vi "Read Configuration.vi"(8 "error in (no error)":errorcluster, 11 "RandomNumberGenerator Controller in":refnum<class "RandomNumberGenerator Controller.lvclass">) -> (0 "error out":errorcluster, 2 "Configuration":T1, 3 "RandomNumberGenerator Controller out":refnum<class "RandomNumberGenerator Controller.lvclass">)   [LabVIEW 2020, in "RandomNumberGenerator.lvlib" / "RandomNumberGenerator Controller.lvclass"]
doc: "<b>Read Configuration</b>\nThis method directly returns the <b>Configuration.ct</b> stored in the class data of this plugin's controller."
uses:
  RandomNumberGenerator Controller.lvclass
  RandomNumberGenerator Controller.lvclass/RandomNumberGenerator Controller.ctl
  PE/Configuration.ctl
  PE/RandomNumberGenerator.lvclass
panel:
  # "#via_ignore"
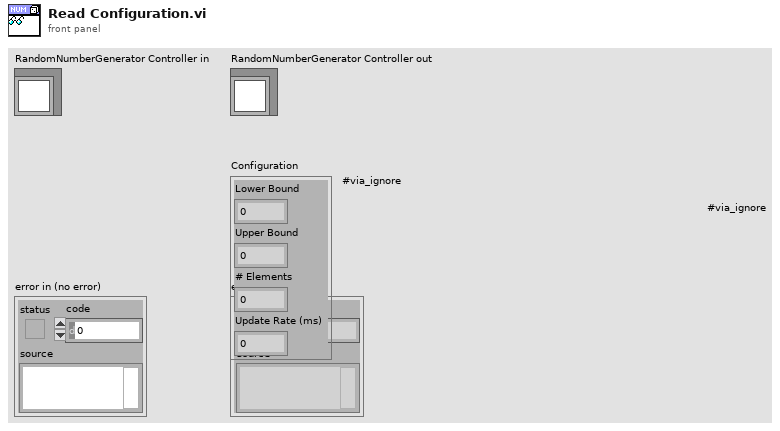
[diagram p1: front panel]
types:
  T1 = typedef "RandomNumberGenerator.lvlib/RandomNumberGenerator.lvclass/Configuration.ctl" = cluster{"Lower Bound":dbl, "Upper Bound":dbl, "# Elements":i32, "Update Rate (ms)":i32}
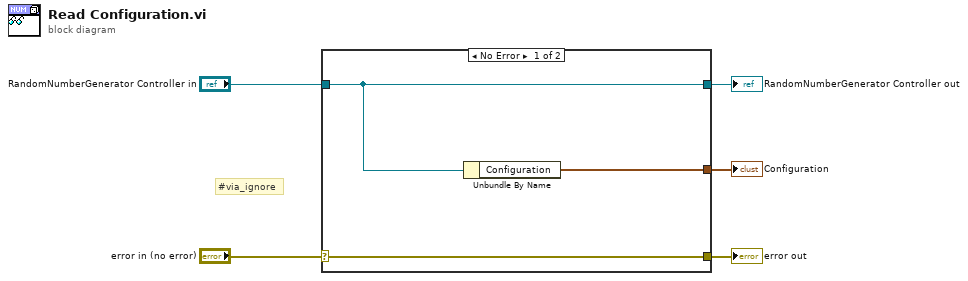
[diagram p0: block diagram]
diagram:
  # "#via_ignore"
  n1 = case shown="No Error" "error in (no error)" {
    selector: "error in (no error)" -> [w8 w9]
    tunnel: [w8 w9] -> w4
    tunnel: [w6 w10] -> w2
    tunnel: "RandomNumberGenerator Controller in" -> [w6 w10]
    tunnel: [w7 _] -> w1
    frame No Error {
      n2 = Unbundle By Name(w6) -> ("Configuration"=w7:T1)
    }
    frame Error {
    }
  }
  "error out" <- w4
  "RandomNumberGenerator Controller out" <- w2
  "Configuration" <- w1
